vi "Edit Control Mode.vi"(8 "Control mode":T2 {"6"."Code"."Data average interval" min=0.0 format="%^#_3g"; "6"."PWM"."Fractional Duty" min=0.0 max=1.0; "5"."Code"."Data average interval" min=0.0 format="%^#_3g"; "5"."PWM"."Fractional Duty" min=0.0 max=1.0; "4"."Code"."Data average interval" min=0.0 format="%^#_3g"; "4"."PWM"."Fractional Duty" min=0.0 max=1.0; "3"."Code"."Data average interval" min=0.0 format="%^#_3g"; "3"."PWM"."Fractional Duty" min=0.0 max=1.0; "2"."Code"."Data average interval" min=0.0 format="%^#_3g"; "2"."PWM"."Fractional Duty" min=0.0 max=1.0; "1"."Code"."Data average interval" min=0.0 format="%^#_3g"; "1"."PWM"."Fractional Duty" min=0.0 max=1.0; "Pump"."Code"."Data average interval" min=0.0 format="%^#_3g"; "Pump"."PWM"."Fractional Duty" min=0.0 max=1.0}, 9 "Switch settings":T7, 10 "Set Points":T9[](array[typedef]) {"value" format="%#_6p"; "variable"."Data average interval" min=0.0 format="%^#_3g"}, 11 "Sensor names":string[](array[string])) -> (0 "Control mode out":T2 {"6"."Code"."Data average interval" min=0.0 format="%^#_3g"; "6"."PWM"."Fractional Duty" min=0.0 max=1.0; "5"."Code"."Data average interval" min=0.0 format="%^#_3g"; "5"."PWM"."Fractional Duty" min=0.0 max=1.0; "4"."Code"."Data average interval" min=0.0 format="%^#_3g"; "4"."PWM"."Fractional Duty" min=0.0 max=1.0; "3"."Code"."Data average interval" min=0.0 format="%^#_3g"; "3"."PWM"."Fractional Duty" min=0.0 max=1.0; "2"."Code"."Data average interval" min=0.0 format="%^#_3g"; "2"."PWM"."Fractional Duty" min=0.0 max=1.0; "1"."Code"."Data average interval" min=0.0 format="%^#_3g"; "1"."PWM"."Fractional Duty" min=0.0 max=1.0; "Pump"."Code"."Data average interval" min=0.0 format="%^#_3g"; "Pump"."PWM"."Fractional Duty" min=0.0 max=1.0}, 1 "Switch settings out":T7)   [LabVIEW 2010]
uses:
  Switch wtih PWM code.ctl
  Switch settings PWM.ctl
  PWM.ctl
  Code.ctl
  Data for Controls.ctl
  Switch control modes.ctl
  type specifier for control code.ctl
  ADT 2/help.ctl
  variable setpoint.ctl
  data ave interval.ctl
panel:
  in  "Help Button":T1
  in  "Cancel Button":bool
  in  "OK Button":bool
  out "code okay":bool[](array[boolean])
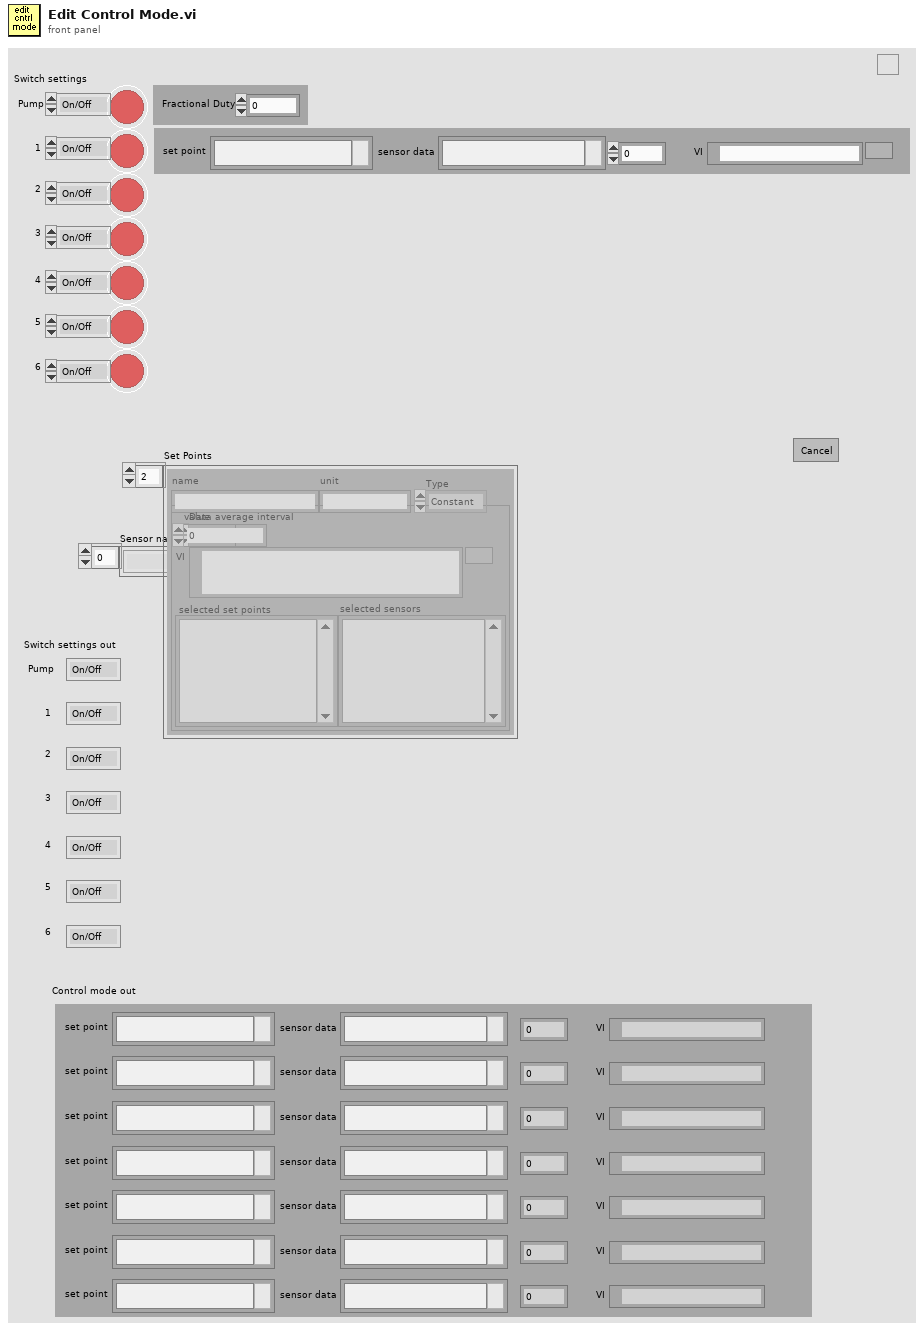
[diagram p1: front panel]
types:
  T1 = typedef "help.ctl" = bool
  T2 = typedef "Switch control modes.ctl" = cluster{"Pump":T3, "1":T3, "2":T3, "3":T3, "4":T3, "5":T3, "6":T3}
  T3 = typedef "Data for Controls.ctl" = cluster{"PWM":T4, "Code":T5}
  T4 = typedef "PWM.ctl" = cluster{"Fractional Duty":dbl}
  T5 = typedef "Code.ctl" = cluster{"set point":i32[], "VI":path, "sensor data":i32[], "Data average interval":dbl, "code ref":T6}
  T6 = typedef "type specifier for control code.ctl" = refnum<vi>
  T7 = typedef "Switch settings PWM.ctl" = cluster{"Pump":T8, "1":T8, "2":T8, "3":T8, "4":T8, "5":T8, "6":T8}
  T8 = typedef "Switch wtih PWM code.ctl" = enum16{"On/Off", "Fraction", "Code"}
  T9 = typedef "variable setpoint.ctl" = cluster{"name":string, "unit":string, "value":dbl, "Type":enum16{"Constant", "Variable"}, "variable":cluster{"selected sensors":i32[], "selected set points":i32[], "VI":path, "Data average interval":T10, "code ref":T6}}
  T10 = typedef "data ave interval.ctl" = dbl
  T11 = cluster{"[0]":T3, "[1]":T3, "[2]":T3, "[3]":T3, "[4]":T3, "[5]":T3, "[6]":T3}
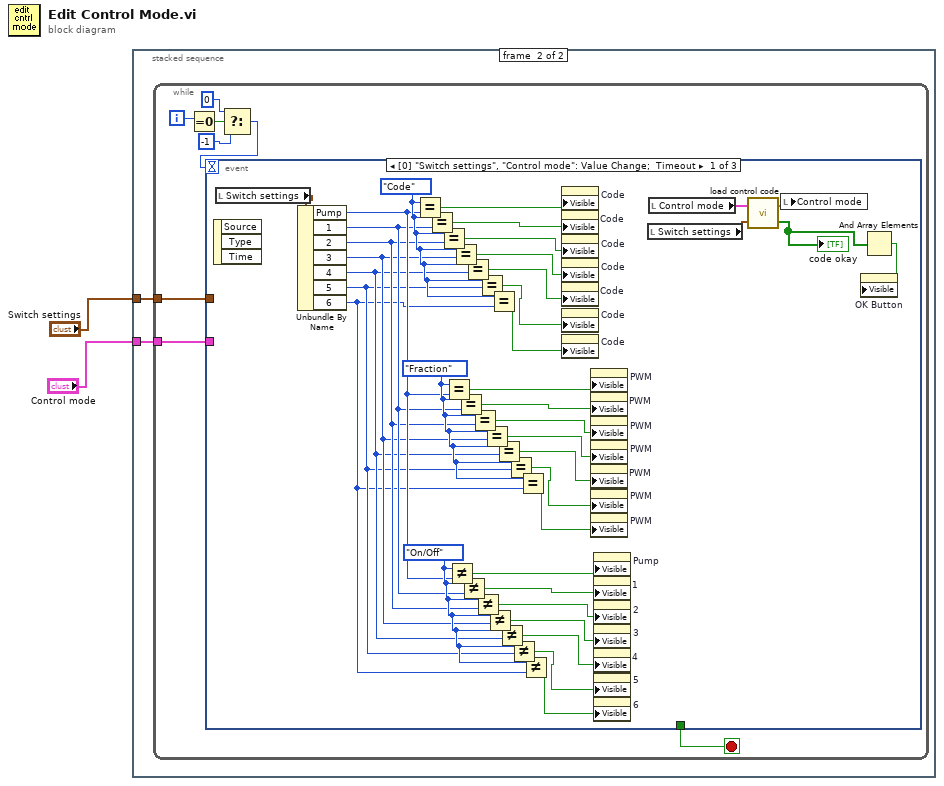
[diagram p0: block diagram]
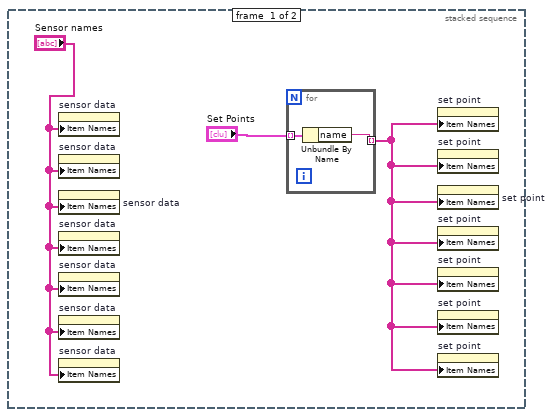
[diagram p2: hidden frame]
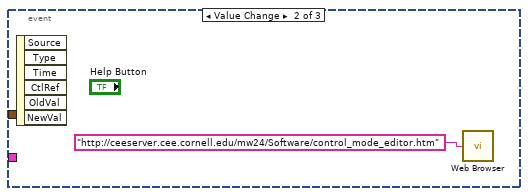
[diagram p3: hidden frame]
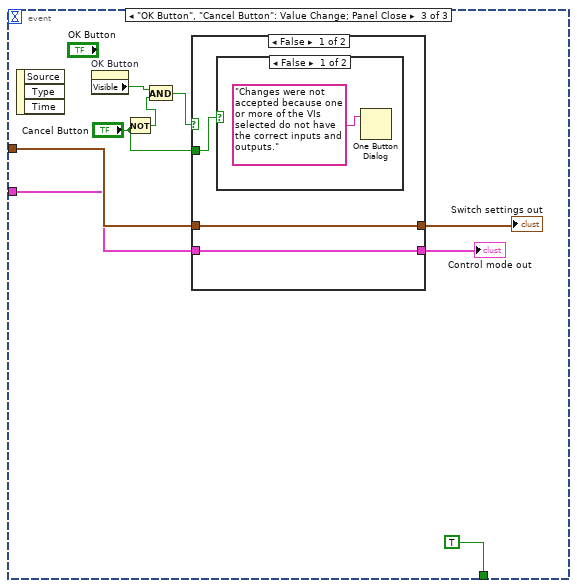
[diagram p4: hidden frame]
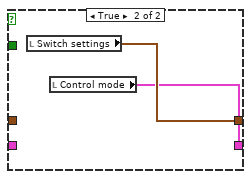
[diagram p6: hidden frame]
diagram:
  n1 = stacked-sequence {
    tunnel: "Switch settings" -> [_ w9]
    tunnel: "Control mode" -> [_ w8]
    frame #0 {
      n2 = property on="sensor data" class="LstBox (strict)"("Item Names"="Sensor names") -> ()  [unwired: 2 in, 2 out]
      n3 = property on="sensor data" class="LstBox (strict)"("Item Names"="Sensor names") -> ()  [unwired: 2 in, 2 out]
      n4 = property on="sensor data" class="LstBox (strict)"("Item Names"="Sensor names") -> ()  [unwired: 2 in, 2 out]
      n5 = property on="sensor data" class="LstBox (strict)"("Item Names"="Sensor names") -> ()  [unwired: 2 in, 2 out]
      n6 = property on="sensor data" class="LstBox (strict)"("Item Names"="Sensor names") -> ()  [unwired: 2 in, 2 out]
      n7 = property on="sensor data" class="LstBox (strict)"("Item Names"="Sensor names") -> ()  [unwired: 2 in, 2 out]
      n8 = property on="sensor data" class="LstBox (strict)"("Item Names"="Sensor names") -> ()  [unwired: 2 in, 2 out]
      n9 = for {
        tunnel: "Set Points" -> [w7] mode=indexing
        tunnel: [w6] -> w4 mode=indexing
        n10 = Unbundle By Name(w7) -> ("name"=w6:string)
      }
      n11 = property on="set point" class="LstBox (strict)"("Item Names"=w4) -> ()  [unwired: 2 in, 2 out]
      n12 = property on="set point" class="LstBox (strict)"("Item Names"=w4) -> ()  [unwired: 2 in, 2 out]
      n13 = property on="set point" class="LstBox (strict)"("Item Names"=w4) -> ()  [unwired: 2 in, 2 out]
      n14 = property on="set point" class="LstBox (strict)"("Item Names"=w4) -> ()  [unwired: 2 in, 2 out]
      n15 = property on="set point" class="LstBox (strict)"("Item Names"=w4) -> ()  [unwired: 2 in, 2 out]
      n16 = property on="set point" class="LstBox (strict)"("Item Names"=w4) -> ()  [unwired: 2 in, 2 out]
      n17 = property on="set point" class="LstBox (strict)"("Item Names"=w4) -> ()  [unwired: 2 in, 2 out]
    }
    frame #1 {
      n18 = while {
        tunnel: w9 -> [w16]
        tunnel: w8 -> [w15]
        i -> [w14]
        stop <- w17 stop-if-true
        n19 = Equal To 0?(x=w14) -> (x = 0?=w13:bool)
        n20 = Select(t=0, s=w13, f=-1) -> (s? t:f=w10:i32)
        n21 = event shown="[0] \"Switch settings\", \"Control mode\": Value Change;  Timeout" {
          selector: _ -> [_ _ _]
          dyn-events: _ -> [_ _ _]
          timeout: w10 -> [_ _ _]
          tunnel: [_ _ TRUE] -> w17
          tunnel: w16 -> [_ _ w62]
          tunnel: w15 -> [_ _ w61]
          event Value Change; Timeout {
            w38 = Switch_wtih_PWM_code."On/Off" ("1")
            w39 = Switch_wtih_PWM_code."Fraction" ("1")
            w54 = Switch_wtih_PWM_code."Code" ("1")
            n22 = event-data() -> ()  [unwired: 1 in, 3 out]
            n23 = local read "Switch settings"() -> (w23:T7)
            n24 = Unbundle By Name(w23) -> ("Pump"=w30:T8, "1"=w29:T8, "2"=w28:T8, "3"=w27:T8, "4"=w26:T8, "5"=w25:T8, "6"=w24:T8)
            n25 = Equal?(x=w54, y=w30) -> (x = y?=w53:bool)
            n26 = Equal?(x=w54, y=w29) -> (x = y?=w52:bool)
            n27 = Equal?(x=w54, y=w28) -> (x = y?=w51:bool)
            n28 = Equal?(x=w39, y=w30) -> (x = y?=w40:bool)
            n29 = Not Equal?(x=w38, y=w30) -> (x != y?=w37:bool)
            n30 = Equal?(x=w54, y=w27) -> (x = y?=w50:bool)
            n31 = Equal?(x=w39, y=w29) -> (x = y?=w41:bool)
            n32 = Not Equal?(x=w38, y=w29) -> (x != y?=w36:bool)
            n33 = Equal?(x=w54, y=w26) -> (x = y?=w49:bool)
            n34 = Equal?(x=w39, y=w28) -> (x = y?=w42:bool)
            n35 = Not Equal?(x=w38, y=w28) -> (x != y?=w35:bool)
            n36 = Equal?(x=w54, y=w25) -> (x = y?=w48:bool)
            n37 = Equal?(x=w39, y=w27) -> (x = y?=w43:bool)
            n38 = Not Equal?(x=w38, y=w27) -> (x != y?=w34:bool)
            n39 = Equal?(x=w54, y=w24) -> (x = y?=w47:bool)
            n40 = Equal?(x=w39, y=w26) -> (x = y?=w44:bool)
            n41 = Not Equal?(x=w38, y=w26) -> (x != y?=w33:bool)
            n42 = Equal?(x=w39, y=w25) -> (x = y?=w45:bool)
            n43 = Not Equal?(x=w38, y=w25) -> (x != y?=w32:bool)
            n44 = Equal?(x=w39, y=w24) -> (x = y?=w46:bool)
            n45 = Not Equal?(x=w38, y=w24) -> (x != y?=w31:bool)
            n46 = property on="Code" class="Clust (strict)"("Visible"=w53) -> ()  [unwired: 2 in, 2 out]
            n47 = property on="Code" class="Clust (strict)"("Visible"=w52) -> ()  [unwired: 2 in, 2 out]
            n48 = property on="Code" class="Clust (strict)"("Visible"=w51) -> ()  [unwired: 2 in, 2 out]
            n49 = property on="Code" class="Clust (strict)"("Visible"=w50) -> ()  [unwired: 2 in, 2 out]
            n50 = property on="Code" class="Clust (strict)"("Visible"=w49) -> ()  [unwired: 2 in, 2 out]
            n51 = property on="Code" class="Clust (strict)"("Visible"=w48) -> ()  [unwired: 2 in, 2 out]
            n52 = property on="Code" class="Clust (strict)"("Visible"=w47) -> ()  [unwired: 2 in, 2 out]
            n53 = property on="PWM" class="Clust (strict)"("Visible"=w40) -> ()  [unwired: 2 in, 2 out]
            n54 = property on="PWM" class="Clust (strict)"("Visible"=w41) -> ()  [unwired: 2 in, 2 out]
            n55 = property on="PWM" class="Clust (strict)"("Visible"=w42) -> ()  [unwired: 2 in, 2 out]
            n56 = property on="PWM" class="Clust (strict)"("Visible"=w43) -> ()  [unwired: 2 in, 2 out]
            n57 = property on="PWM" class="Clust (strict)"("Visible"=w44) -> ()  [unwired: 2 in, 2 out]
            n58 = property on="PWM" class="Clust (strict)"("Visible"=w45) -> ()  [unwired: 2 in, 2 out]
            n59 = property on="PWM" class="Clust (strict)"("Visible"=w46) -> ()  [unwired: 2 in, 2 out]
            n60 = property on="Pump" class="Clust (strict)"("Visible"=w37) -> ()  [unwired: 2 in, 2 out]
            n61 = property on="1" class="Clust (strict)"("Visible"=w36) -> ()  [unwired: 2 in, 2 out]
            n62 = property on="2" class="Clust (strict)"("Visible"=w35) -> ()  [unwired: 2 in, 2 out]
            n63 = property on="3" class="Clust (strict)"("Visible"=w34) -> ()  [unwired: 2 in, 2 out]
            n64 = property on="4" class="Clust (strict)"("Visible"=w33) -> ()  [unwired: 2 in, 2 out]
            n65 = property on="5" class="Clust (strict)"("Visible"=w32) -> ()  [unwired: 2 in, 2 out]
            n66 = property on="6" class="Clust (strict)"("Visible"=w31) -> ()  [unwired: 2 in, 2 out]
            n67 = local read "Switch settings"() -> (w19:T7)
            n68 = local read "Control mode"() -> (w21:T2)
            n69 = call "load control code.vi"("Switch settings"=w19, "Control mode"=w21) -> ("code okay"=w18:bool[], "Control mode out"=w20:T11)
            "code okay" <- w18
            n70 = local write "Control mode"(w20) -> ()
            n71 = And Array Elements(Boolean array=w18) -> (logical AND=w22:bool)
            n72 = property on="OK Button" class="Bool"("Visible"=w22) -> ()  [unwired: 2 in, 2 out]
          }
          event Value Change {
            n73 = event-data() -> ()  [unwired: 1 in, 6 out]
            n74 = call "Web Browser.vi"("URL"="http://ceeserver.cee.cornell.edu/mw24/Software/control_mode_editor.htm") -> ()  [unwired: 1 in]
          }
          event "OK Button", "Cancel Button": Value Change; Panel Close {
            n75 = event-data() -> ()  [unwired: 1 in, 3 out]
            n76 = property on="OK Button" class="Bool"() -> ("Visible"=w57:bool)  [unwired: 2 in, 2 out]
            n77 = Not(x="Cancel Button") -> (.not. x?=w59:bool)
            n78 = And(x=w57, y=w59) -> (x .and. y?=w58:bool)
            n79 = case shown="False" w58 {
              tunnel: [w67 w70] -> w63
              tunnel: w62 -> [w67 _]
              tunnel: w61 -> [w66 _]
              tunnel: [w66 w69] -> w60
              tunnel: "Cancel Button" -> [w65 _]
              frame False {
                n80 = case shown="False" w65 {
                  frame False {
                    n81 = One Button Dialog(message="Changes were not accepted because one or more of the VIs selected do not have the correct inputs and outputs.") -> ()  [unwired: 1 in, 1 out]
                  }
                  frame True {
                  }
                }
              }
              frame True {
                n82 = local read "Switch settings"() -> (w70:T7)
                n83 = local read "Control mode"() -> (w69:T2)
              }
            }
            "Switch settings out" <- w63
            "Control mode out" <- w60
          }
        }
      }
    }
  }
